vi "T1005V1.vi"() -> ()   [LabVIEW 2016]
uses:
  <vilib>/Instr/_visa.llb/VISA Configure Serial Port (Instr).vi
panel:
  out "接收命令":string
  out "输入命令":string
  in  "复位":bool
  in  "暂停":bool
  in  "小数":string
  in  "卡滞发生时间":string
  in  "角度（小数）":string
  in  "卡滞角度":string
  in  "退化故障":string(combo)
  in  "控制方法":string(combo)
  in  "波特率":dbl
  in  "故障腿":string(combo)
  in  "data bits (8)":u16=8 caption="数据比特(8)" min=5 max=8 step=1
  in  "arduino端口":refnum<visa-resource-name>
  in  "控制程序启动":bool
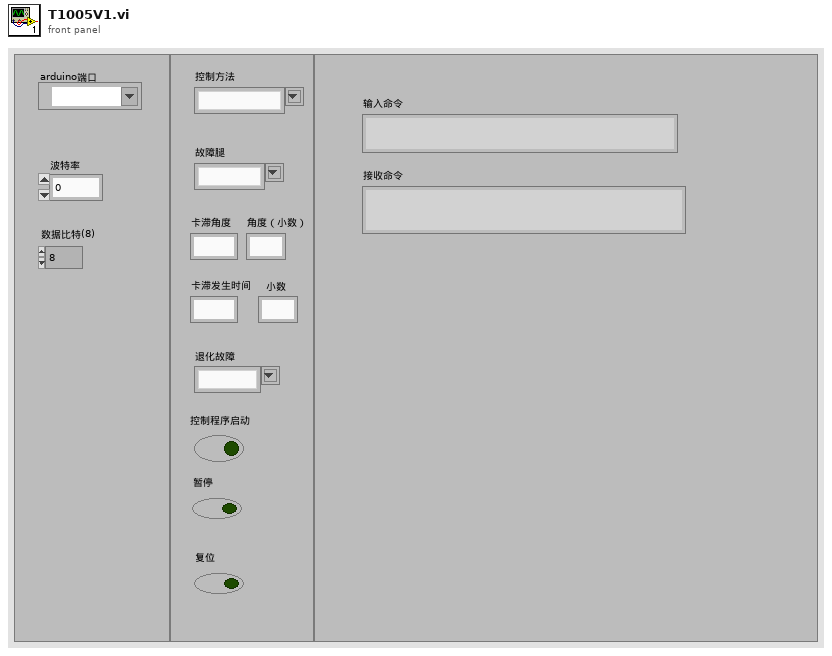
[diagram p1: front panel]
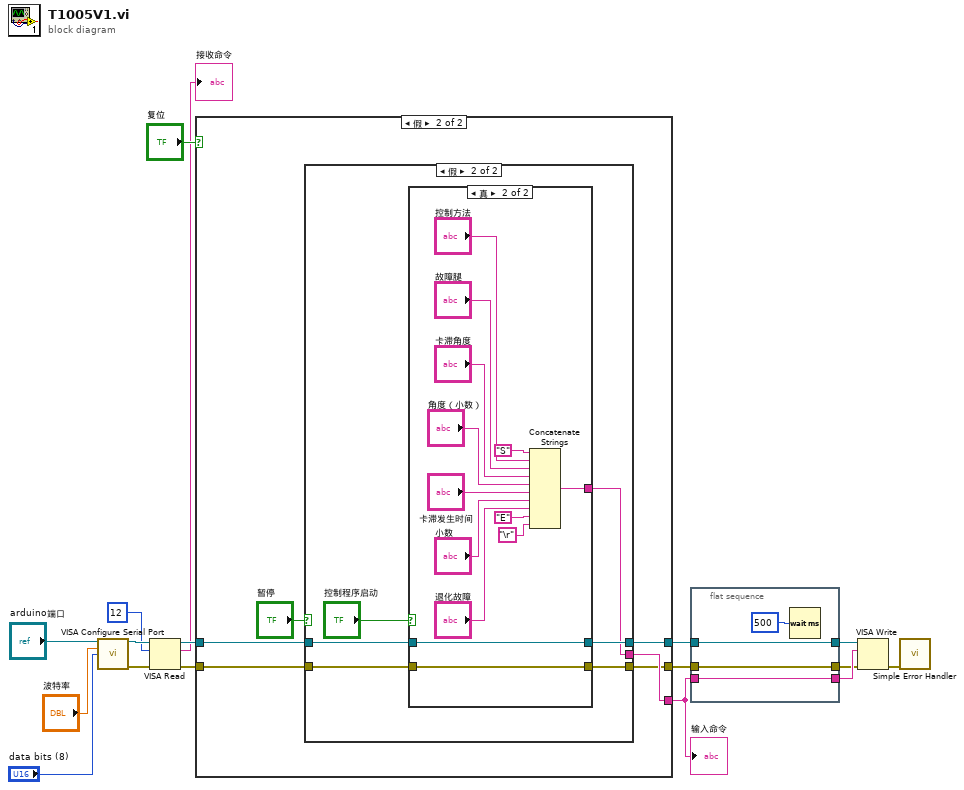
[diagram p0: block diagram]
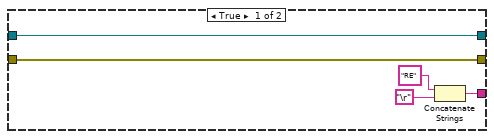
[diagram p2: hidden frame]
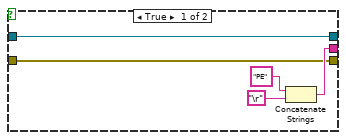
[diagram p3: hidden frame]
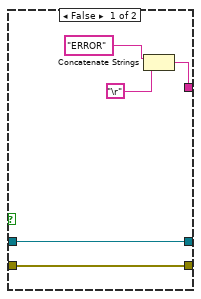
[diagram p4: hidden frame]
diagram:
  n1 = call-poly "VISA Configure Serial Port"("VISA resource name"="arduino端口", "baud rate (9600)"="波特率", "data bits (8)"="data bits (8)") -> ("VISA resource name out"=w14:refnum<visa-resource-name>, "error out"=w11:errorcluster)  [unwired: 11 in]
  n2 = VISA Read(VISA resource name=w14, byte count=12, error in (no error)=w11) -> (VISA resource name out=w12:refnum<visa-resource-name>, read buffer=→"接收命令":string, error out=w9:errorcluster)  [unwired: 1 out]
  n3 = case shown="假" "复位" {
    tunnel: w12 -> [w18 w28]
    tunnel: w9 -> [w19 w27]
    tunnel: [w18 w25] -> w6
    tunnel: [w20 w24] -> w5
    tunnel: [w19 w23] -> w4
    frame True {
      n4 = Concatenate Strings("RE", "\r") -> (w20:string)
    }
    frame False {
      n5 = case shown="假" "暂停" {
        tunnel: w28 -> [w31 w39]
        tunnel: w27 -> [w29 w37]
        tunnel: [w31 w36] -> w25
        tunnel: [w30 w35] -> w24
        tunnel: [w29 w34] -> w23
        frame True {
          n6 = Concatenate Strings("PE", "\r") -> (w30:string)
        }
        frame False {
          n7 = case shown="真" "控制程序启动" {
            tunnel: w39 -> [w43 w47]
            tunnel: w37 -> [w44 w45]
            tunnel: [w43 w47] -> w36
            tunnel: [w41 w46] -> w35
            tunnel: [w44 w45] -> w34
            frame False {
              n8 = Concatenate Strings("ERROR", "\r") -> (w41:string)
            }
            frame True {
              n9 = Concatenate Strings("S", "控制方法", "故障腿", "卡滞角度", "角度（小数）", "卡滞发生时间", "小数", "退化故障", "E", "\r") -> (w46:string)
            }
          }
        }
      }
    }
  }
  "输入命令" <- w5
  n10 = flat-sequence {
    tunnel: w6 -> [w60]
    tunnel: w5 -> [w59]
    tunnel: w4 -> [w58]
    tunnel: [w60] -> w3
    tunnel: [w59] -> w2
    tunnel: [w58] -> w1
    frame #0 {
      n11 = Wait (ms)(milliseconds to wait=500) -> ()  [unwired: 1 out]
    }
  }
  n12 = VISA Write(VISA resource name=w3, write buffer=w2, error in (no error)=w1) -> (error out=w7:errorcluster)  [unwired: 2 out]
  n13 = call <vilib>:"Simple Error Handler.vi"("error in (no error)"=w7) -> ()  [unwired: 1 in, 8 out]
